vi "ma_Reconstruct detected signals.vi"(9 "dt":dbl, 10 "# samples":i32, 11 "multiple tone information":T1(array[cluster]) {"detected phase (deg)" format="%.2p"; "detected amplitude" format="%.2p"; "detected frequency" format="%.2p"}) -> (2 "detected Hann spectrum":cdb[](array[numeric]), 3 "detected time array":dbl[](array[numeric]))   [LabVIEW 2020, in "NI_MAPro.lvlib"]
uses:
  NI_MAPro.lvlib
  NI_AALBase.lvlib
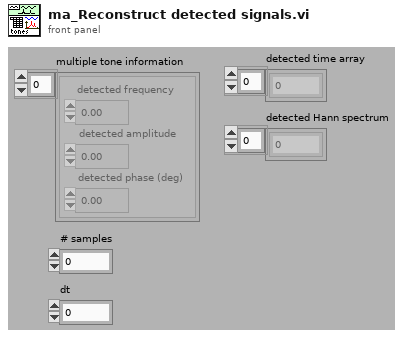
[diagram p1: front panel]
types:
  T1 = cluster{"detected frequency":dbl, "detected amplitude":dbl, "detected phase (deg)":dbl}[]
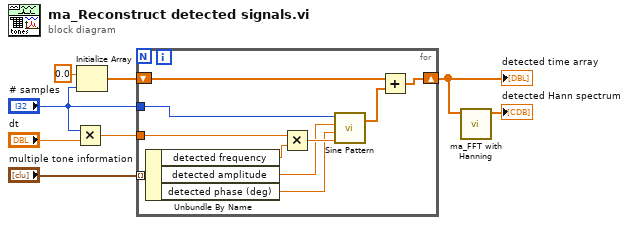
[diagram p0: block diagram]
diagram:
  n1 = Multiply(x="# samples", y="dt") -> (x*y=w6:dbl)
  n2 = Initialize Array(0.0, "# samples") -> (w5:dbl[])
  n3 = for {
    tunnel: "multiple tone information" -> [w18] mode=indexing
    tunnel: "# samples" -> [w17]
    tunnel: w6 -> [w14]
    shift-right: [w9] -> w2
    shift-left: w5 -> [w10]
    n4 = Unbundle By Name(w18) -> ("detected frequency"=w15:dbl, "detected amplitude"=w13:dbl, "detected phase (deg)"=w12:dbl)
    n5 = Multiply(x=w14, y=w15) -> (x*y=w16:dbl)
    n6 = call "Sine Pattern.vi"("cycles"=w16, "phase(degrees)"=w12, "amplitude"=w13, "samples"=w17) -> ("Sinusoidal Pattern"=w11:dbl[])  [unwired: 1 out]
    n7 = Add(x=w10, y=w11) -> (x+y=w9:dbl[])
  }
  "detected time array" <- w2
  n8 = call "ma_FFT with Hanning.vi"("time signal data"=w2) -> ("complex Hann spectrum"=→"detected Hann spectrum":cdb[])  [unwired: 2 in, 8 out]
